vi "1553B_帧解析_v4_21.vi"(8 "Register name":string="Zhufen_period", 9 "Counter":u64, 11 "数组":u8[](array[numeric])) -> (1 "连接的字符串":string, 3 "输出簇":T1)   [LabVIEW 2012]
uses:
  <vilib>/GPower/VIRegister/Library/Convert/ToU16.vi
  <vilib>/GPower/VIRegister/Library/SubVIs/FindRegisterData.vi
  <vilib>/GPower/VIRegister/Library/SubVIs/ReadSub.vi
  <vilib>/GPower/VIRegister/Library/QManager/GetRegisterData.vi
  <vilib>/GPower/Error/Library/SetError.vi
  <vilib>/GPower/Error/Library/FilterCodes.vi
  <vilib>/GPower/Error/Library/Filter/FilterMulti.vi
  <vilib>/GPower/VIRegister/Library/QManager/QManagerAction.vi
  <vilib>/GPower/Error/Library/ErrorType.vi
  <vilib>/GPower/Error/Library/SplitAppended.vi
  <vilib>/GPower/Error/Library/SubVIs/ExplanationToError.vi
  <vilib>/GPower/VIRegister/Library/QManager/GetQName.vi
  <vilib>/GPower/VIRegister/Library/QManager/StartQManager.vi
  <vilib>/Utility/error.llb/Trim Whitespace.vi
  <vilib>/dlg_ctls.llb/Space Constant.vi
  <vilib>/Utility/error.llb/Error Code Database.vi
  <vilib>/GPower/Error/Library/SubVIs/SetStatus.vi
  <vilib>/GPower/Error/Library/AppendErrors.vi
  <vilib>/GPower/Error/Library/Append/AppendSingle.vi
  <vilib>/GPower/VIRegister/VIRegister.lvlib
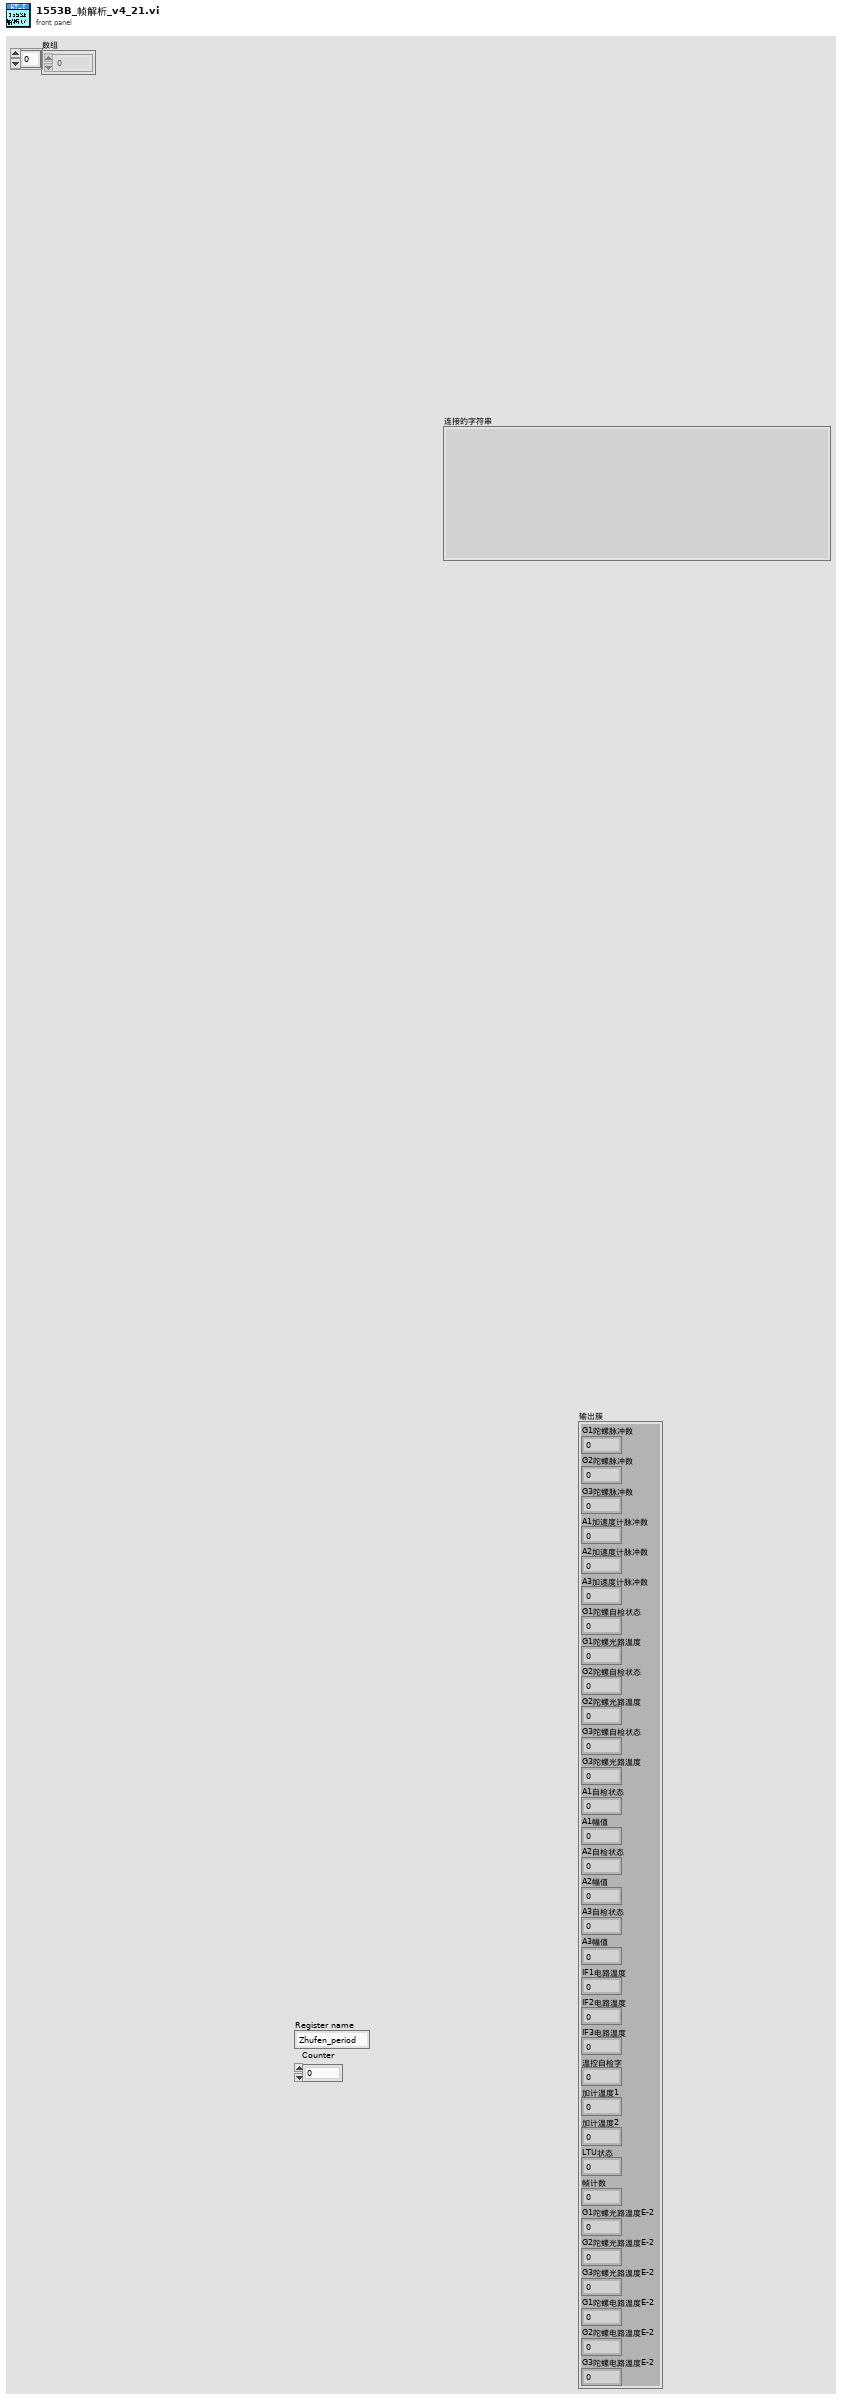
[diagram p1: front panel]
types:
  T1 = cluster{"G1陀螺脉冲数":i32, "G2陀螺脉冲数":i32, "G3陀螺脉冲数":i32, "A1加速度计脉冲数":i16, "A2加速度计脉冲数":i16, "A3加速度计脉冲数":i16, "G1陀螺自检状态":u8, "G1陀螺光路温度":i8, "G2陀螺自检状态":u8, "G2陀螺光路温度":i8, "G3陀螺自检状态":u8, "G3陀螺光路温度":i8, "A1自检状态":u8, "A1幅值":u8, "A2自检状态":u8, "A2幅值":u8, "A3自检状态":u8, "A3幅值":u8, "IF1电路温度":i8, "IF2电路温度":i8, "IF3电路温度":i8, "温控自检字":u8, "加计温度1":i16, "加计温度2":i16, "LTU状态":u8, "帧计数":u8, "G1陀螺光路温度E-2":i16, "G2陀螺光路温度E-2":i16, "G3陀螺光路温度E-2":i16, "G1陀螺电路温度E-2":i16, "G2陀螺电路温度E-2":i16, "G3陀螺电路温度E-2":i16}
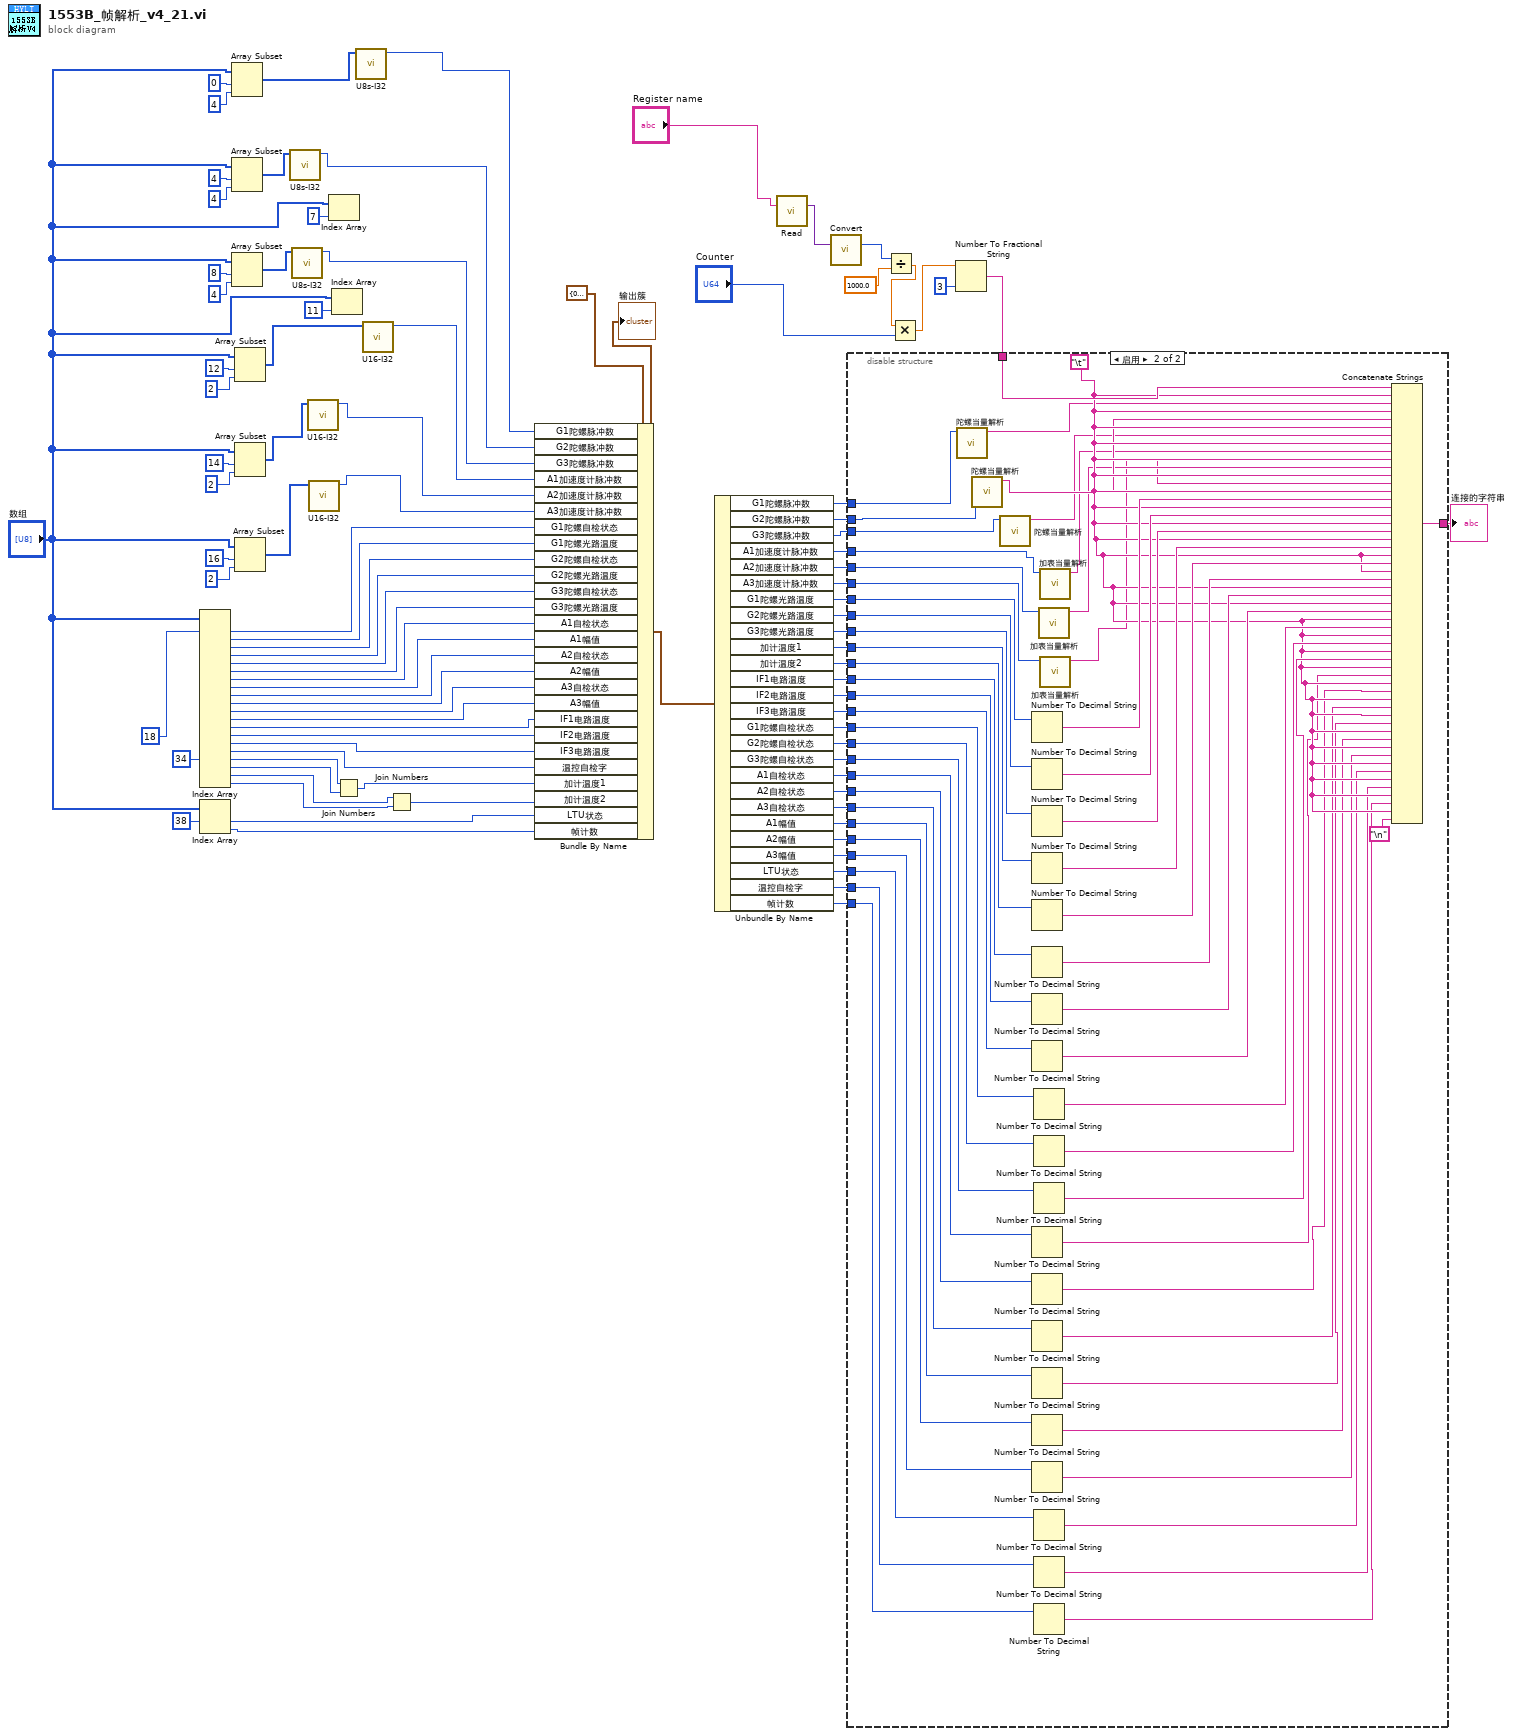
[diagram p0: block diagram]
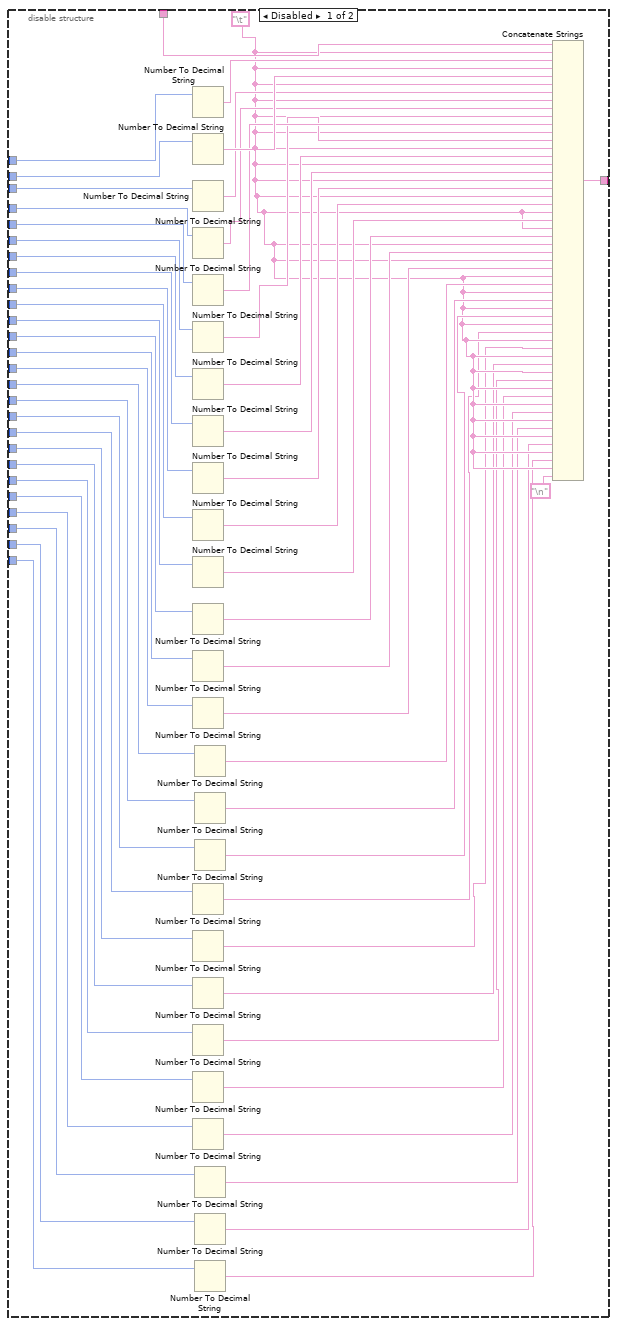
[diagram p2: hidden frame]
diagram:
  n1 = Index Array(array="数组", index #1=18 ("索引"), index #17=34 ("索引")) -> (element #1=w79:u8, element #2=w38:u8, element #3=w78:u8, element #4=w77:u8, element #5=w37:u8, element #6=w36:u8, element #7=w35:u8, element #8=w34:u8, element #9=w33:u8, element #10=w32:u8, element #11=w31:u8, element #12=w30:u8, element #13=w29:u8, element #14=w28:u8, element #15=w27:u8, element #16=w26:u8, element #17=w25:u8, element #18=w23:u8, element #19=w21:u8, element #20=w20:u8)  [unwired: 18 in]
  n2 = Index Array(array="数组", index #1=38 ("索引")) -> (element #1=w17:u8, element #2=w6:u8)  [unwired: 1 in]
  n3 = Array Subset(array="数组", index=0 ("索引"), length=u8 4 ("新元素/子数组")) -> (w74:u8[])
  n4 = Array Subset(array="数组", index=4 ("索引"), length=u8 4 ("新元素/子数组")) -> (w72:u8[])
  n5 = Array Subset(array="数组", index=8 ("索引"), length=u8 4 ("新元素/子数组")) -> (w69:u8[])
  n6 = Array Subset(array="数组", index=12 ("索引"), length=u8 2 ("新元素/子数组")) -> (w68:u8[])
  n7 = Array Subset(array="数组", index=14 ("索引"), length=u8 2 ("新元素/子数组")) -> (w66:u8[])
  n8 = Array Subset(array="数组", index=16 ("索引"), length=u8 2 ("新元素/子数组")) -> (w64:u8[])
  n9 = call "U8s-I32.vi"("数组"=w72) -> ("I32转换"=w71:i32)  [unwired: 10 in]
  n10 = call "U8s-I32.vi"("数组"=w69) -> ("I32转换"=w70:i32)  [unwired: 10 in]
  n11 = call "U16-I32.vi"("数组"=w66) -> ("I32转换"=w65:i16)  [unwired: 10 in]
  n12 = call "U16-I32.vi"("数组"=w64) -> ("I32转换"=w63:i16)  [unwired: 10 in]
  n13 = Index Array(array="数组", index=7 ("索引")) -> ()  [unwired: 1 out]
  n14 = Index Array(array="数组", index=11 ("索引")) -> ()  [unwired: 1 out]
  n15 = Join Numbers(hi=w25, lo=w23) -> ((hi.lo)=w24:u16)
  n16 = call "U8s-I32.vi"("数组"=w74) -> ("I32转换"=w73:i32)  [unwired: 10 in]
  n17 = call "U16-I32.vi"("数组"=w68) -> ("I32转换"=w67:i16)  [unwired: 10 in]
  n18 = Join Numbers(hi=w21, lo=w20) -> ((hi.lo)=w22:u16)
  n19 = Bundle By Name(cluster=T1 {"G1陀螺脉冲数"=0, "G2陀螺脉冲数"=0, "G3陀螺脉冲数"=0, "A1加速度计脉冲数"=0, "A2加速度计脉冲数"=0, "A3加速度计脉冲数"=0, "G1陀螺自检状态"=0, "G1陀螺光路温度"=0, "G2陀螺自检状态"=0, "G2陀螺光路温度"=0, "G3陀螺自检状态"=0, "G3陀螺光路温度"=0, "A1自检状态"=0, "A1幅值"=0, "A2自检状态"=0, "A2幅值"=0, "A3自检状态"=0, "A3幅值"=0, "IF1电路温度"=0, "IF2电路温度"=0, "IF3电路温度"=0, "温控自检字"=0, "加计温度1"=0, "加计温度2"=0, "LTU状态"=0, "帧计数"=0, "G1陀螺光路温度E-2"=0, "G2陀螺光路温度E-2"=0, "G3陀螺光路温度E-2"=0, "G1陀螺电路温度E-2"=0, "G2陀螺电路温度E-2"=0, "G3陀螺电路温度E-2"=0} ("输入簇"), "G1陀螺脉冲数"=w73, "G2陀螺脉冲数"=w71, "G3陀螺脉冲数"=w70, "A1加速度计脉冲数"=w67, "A2加速度计脉冲数"=w65, "A3加速度计脉冲数"=w63, "G1陀螺自检状态"=w79, "G1陀螺光路温度"=w38, "G2陀螺自检状态"=w78, "G2陀螺光路温度"=w77, "G3陀螺自检状态"=w37, "G3陀螺光路温度"=w36, "A1自检状态"=w35, "A1幅值"=w34, "A2自检状态"=w33, "A2幅值"=w32, "A3自检状态"=w31, "A3幅值"=w30, "IF1电路温度"=w29, "IF2电路温度"=w28, "IF3电路温度"=w27, "温控自检字"=w26, "加计温度1"=w24, "加计温度2"=w22, "LTU状态"=w17, "帧计数"=w6) -> (w4:T1)
  "输出簇" <- w4
  n20 = Unbundle By Name(w4) -> ("G1陀螺脉冲数"=w1:i32, "G2陀螺脉冲数"=w62:i32, "G3陀螺脉冲数"=w61:i32, "A1加速度计脉冲数"=w60:i16, "A2加速度计脉冲数"=w59:i16, "A3加速度计脉冲数"=w58:i16, "G1陀螺光路温度"=w57:i8, "G2陀螺光路温度"=w56:i8, "G3陀螺光路温度"=w55:i8, "加计温度1"=w54:i16, "加计温度2"=w53:i16, "IF1电路温度"=w52:i8, "IF2电路温度"=w51:i8, "IF3电路温度"=w50:i8, "G1陀螺自检状态"=w43:u8, "G2陀螺自检状态"=w42:u8, "G3陀螺自检状态"=w41:u8, "A1自检状态"=w16:u8, "A2自检状态"=w15:u8, "A3自检状态"=w14:u8, "A1幅值"=w13:u8, "A2幅值"=w12:u8, "A3幅值"=w11:u8, "LTU状态"=w10:u8, "温控自检字"=w9:u8, "帧计数"=w8:u8)
  n21 = call <vilib>:"Read.vi"("Register name"="Register name") -> ("Register value"=w40:variant)  [unwired: 11 in, 3 out]
  n22 = call-poly <vilib>:"Convert.vi"("Register value in"=w40) -> ("Register value out"=w39:u16)  [unwired: 13 in, 1 out]
  n23 = Divide(x=w39, y=sgl 1000.0) -> (x/y=w45:sgl)
  n24 = Multiply(x=w45, y="Counter") -> (x*y=w44:sgl)
  n25 = Number To Fractional String(number=w44, precision (6)=i16 3 ("精度(6)")) -> (F-format string=w46:string)  [unwired: 2 in]
  n26 = disable-structure shown="启用" {
    disable-tunnel: w62 -> [w148 w158]
    disable-tunnel: w61 -> [w147 w156]
    disable-tunnel: w60 -> [w146 w154]
    disable-tunnel: w59 -> [w145 w151]
    disable-tunnel: w58 -> [w144 w150]
    disable-tunnel: w57 -> [w143 w204]
    disable-tunnel: w56 -> [w142 w203]
    disable-tunnel: w55 -> [w141 w202]
    disable-tunnel: w54 -> [w140 w201]
    disable-tunnel: w53 -> [w139 w200]
    disable-tunnel: w52 -> [w138 w199]
    disable-tunnel: w51 -> [w137 w198]
    disable-tunnel: w50 -> [w136 w197]
    disable-tunnel: [w121 w188] -> w49
    disable-tunnel: w46 -> [w120 w187]
    disable-tunnel: w43 -> [w119 w186]
    disable-tunnel: w42 -> [w118 w185]
    disable-tunnel: w41 -> [w117 w184]
    disable-tunnel: w16 -> [w113 w180]
    disable-tunnel: w15 -> [w112 w179]
    disable-tunnel: w14 -> [w111 w178]
    disable-tunnel: w13 -> [w110 w177]
    disable-tunnel: w12 -> [w109 w176]
    disable-tunnel: w11 -> [w108 w175]
    disable-tunnel: w10 -> [w107 w174]
    disable-tunnel: w9 -> [w106 w173]
    disable-tunnel: w8 -> [w105 w172]
    disable-tunnel: w1 -> [w93 w160]
    frame Disabled {
      w104 = "\t"
      n27 = Number To Decimal String(number=w93) -> (decimal integer string=w135:string)  [unwired: 1 in]
      n28 = Number To Decimal String(number=w148) -> (decimal integer string=w134:string)  [unwired: 1 in]
      n29 = Number To Decimal String(number=w147) -> (decimal integer string=w133:string)  [unwired: 1 in]
      n30 = Number To Decimal String(number=w146) -> (decimal integer string=w132:string)  [unwired: 1 in]
      n31 = Number To Decimal String(number=w145) -> (decimal integer string=w131:string)  [unwired: 1 in]
      n32 = Number To Decimal String(number=w144) -> (decimal integer string=w130:string)  [unwired: 1 in]
      n33 = Number To Decimal String(number=w143) -> (decimal integer string=w129:string)  [unwired: 1 in]
      n34 = Number To Decimal String(number=w142) -> (decimal integer string=w128:string)  [unwired: 1 in]
      n35 = Number To Decimal String(number=w141) -> (decimal integer string=w127:string)  [unwired: 1 in]
      n36 = Number To Decimal String(number=w140) -> (decimal integer string=w126:string)  [unwired: 1 in]
      n37 = Number To Decimal String(number=w139) -> (decimal integer string=w125:string)  [unwired: 1 in]
      n38 = Number To Decimal String(number=w138) -> (decimal integer string=w124:string)  [unwired: 1 in]
      n39 = Number To Decimal String(number=w137) -> (decimal integer string=w123:string)  [unwired: 1 in]
      n40 = Number To Decimal String(number=w136) -> (decimal integer string=w122:string)  [unwired: 1 in]
      n41 = Number To Decimal String(number=w113) -> (decimal integer string=w103:string)  [unwired: 1 in]
      n42 = Number To Decimal String(number=w112) -> (decimal integer string=w102:string)  [unwired: 1 in]
      n43 = Number To Decimal String(number=w111) -> (decimal integer string=w101:string)  [unwired: 1 in]
      n44 = Number To Decimal String(number=w110) -> (decimal integer string=w100:string)  [unwired: 1 in]
      n45 = Number To Decimal String(number=w109) -> (decimal integer string=w99:string)  [unwired: 1 in]
      n46 = Number To Decimal String(number=w108) -> (decimal integer string=w98:string)  [unwired: 1 in]
      n47 = Number To Decimal String(number=w119) -> (decimal integer string=w116:string)  [unwired: 1 in]
      n48 = Number To Decimal String(number=w118) -> (decimal integer string=w115:string)  [unwired: 1 in]
      n49 = Number To Decimal String(number=w117) -> (decimal integer string=w114:string)  [unwired: 1 in]
      n50 = Number To Decimal String(number=w107) -> (decimal integer string=w97:string)  [unwired: 1 in]
      n51 = Number To Decimal String(number=w106) -> (decimal integer string=w96:string)  [unwired: 1 in]
      n52 = Number To Decimal String(number=w105) -> (decimal integer string=w95:string)  [unwired: 1 in]
      n53 = Concatenate Strings(w120, w104, w135, w104, w134, w104, w133, w104, w132, w104, w131, w104, w130, w104, w129, w104, w128, w104, w127, w104, w126, w104, w125, w104, w124, w104, w123, w104, w122, w104, w116, w104, w115, w104, w114, w104, w103, w104, w102, w104, w101, w104, w100, w104, w99, w104, w98, w104, w97, w104, w96, w104, w95, w104, "\n") -> (w121:string)
    }
    frame Enabled {
      w171 = "\t"
      n54 = call "陀螺当量解析.vi"("输入"=w160) -> ("输出"=w159:string)  [unwired: 9 in, 1 out]
      n55 = call "陀螺当量解析.vi"("输入"=w158) -> ("输出"=w157:string)  [unwired: 9 in, 1 out]
      n56 = call "陀螺当量解析.vi"("输入"=w156) -> ("输出"=w155:string)  [unwired: 9 in, 1 out]
      n57 = Number To Decimal String(number=w204) -> (decimal integer string=w196:string)  [unwired: 1 in]
      n58 = Number To Decimal String(number=w203) -> (decimal integer string=w195:string)  [unwired: 1 in]
      n59 = Number To Decimal String(number=w202) -> (decimal integer string=w194:string)  [unwired: 1 in]
      n60 = Number To Decimal String(number=w201) -> (decimal integer string=w193:string)  [unwired: 1 in]
      n61 = Number To Decimal String(number=w200) -> (decimal integer string=w192:string)  [unwired: 1 in]
      n62 = Number To Decimal String(number=w199) -> (decimal integer string=w191:string)  [unwired: 1 in]
      n63 = Number To Decimal String(number=w198) -> (decimal integer string=w190:string)  [unwired: 1 in]
      n64 = Number To Decimal String(number=w197) -> (decimal integer string=w189:string)  [unwired: 1 in]
      n65 = Number To Decimal String(number=w180) -> (decimal integer string=w170:string)  [unwired: 1 in]
      n66 = Number To Decimal String(number=w179) -> (decimal integer string=w169:string)  [unwired: 1 in]
      n67 = Number To Decimal String(number=w178) -> (decimal integer string=w168:string)  [unwired: 1 in]
      n68 = Number To Decimal String(number=w177) -> (decimal integer string=w167:string)  [unwired: 1 in]
      n69 = Number To Decimal String(number=w176) -> (decimal integer string=w166:string)  [unwired: 1 in]
      n70 = Number To Decimal String(number=w175) -> (decimal integer string=w165:string)  [unwired: 1 in]
      n71 = Number To Decimal String(number=w186) -> (decimal integer string=w183:string)  [unwired: 1 in]
      n72 = Number To Decimal String(number=w185) -> (decimal integer string=w182:string)  [unwired: 1 in]
      n73 = Number To Decimal String(number=w184) -> (decimal integer string=w181:string)  [unwired: 1 in]
      n74 = Number To Decimal String(number=w174) -> (decimal integer string=w164:string)  [unwired: 1 in]
      n75 = Number To Decimal String(number=w173) -> (decimal integer string=w163:string)  [unwired: 1 in]
      n76 = Number To Decimal String(number=w172) -> (decimal integer string=w162:string)  [unwired: 1 in]
      n77 = call "加表当量解析.vi"("输入"=w151) -> ("输出"=w152:string)  [unwired: 9 in, 1 out]
      n78 = call "加表当量解析.vi"("输入"=w154) -> ("输出"=w153:string)  [unwired: 9 in, 1 out]
      n79 = call "加表当量解析.vi"("输入"=w150) -> ("输出"=w149:string)  [unwired: 9 in, 1 out]
      n80 = Concatenate Strings(w187, w171, w159, w171, w157, w171, w155, w171, w153, w171, w152, w171, w149, w171, w196, w171, w195, w171, w194, w171, w193, w171, w192, w171, w191, w171, w190, w171, w189, w171, w183, w171, w182, w171, w181, w171, w170, w171, w169, w171, w168, w171, w167, w171, w166, w171, w165, w171, w164, w171, w163, w171, w162, w171, "\n") -> (w188:string)
    }
  }
  "连接的字符串" <- w49
